vi "Write.vi"(8 "error in (no error)":errorcluster, 9 "Cell (Append to next row)":cluster{"Row":i32, "Col":i32}={"Row"=-1, "Col"=-1}, 10 "Data":variant, 11 "Excel in":refnum<class "Excel.lvclass">) -> (0 "error out":errorcluster, 3 "Excel out":refnum<class "Excel.lvclass">)   [LabVIEW 2016, in "Excel.lvclass"]
doc: "Writes Data to the active worksheet referenced in the Excel input object.\n\nIf a cell is specified and Data is a singleton the data will be written to that cell. \nIf a cell is specified and Data is 1D the data will be written beginning at that cell and continuing rightwards.\nIf a cell is specified and Data is 2D the data will be written as a matrix with it's first (top left) element beginning in that cell. The data will be formatted as it appears in LabVIEW (i.e. no transposition required).\n\nIf cell is not specified Data will be written starting from column A in the first available row following the rules outlined above.\n\nData cannot have dimension higher than 2."
uses:
  Excel.lvclass
  Excel.lvclass/Excel.ctl
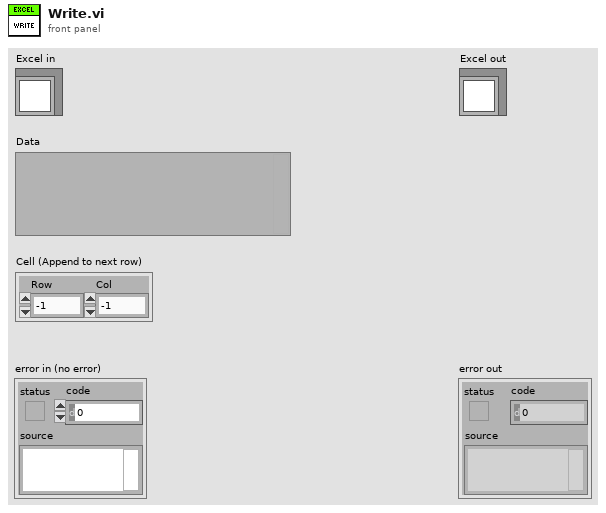
[diagram p1: front panel]
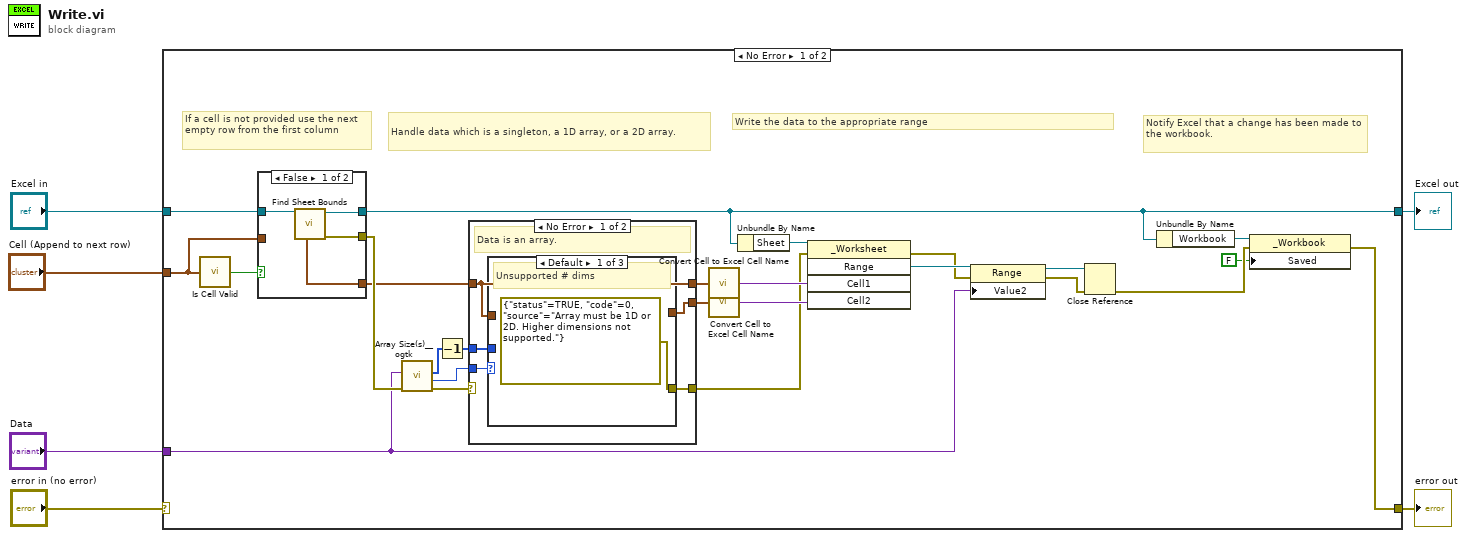
[diagram p0: block diagram]
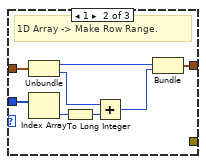
[diagram p2: hidden frame]
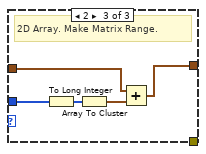
[diagram p3: hidden frame]
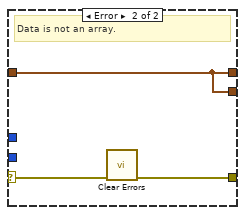
[diagram p4: hidden frame]
diagram:
  n1 = case shown="No Error" "error in (no error)" {
    selector: "error in (no error)" -> [_ w61]
    tunnel: [w7 w61] -> w5
    tunnel: [w10 w60] -> w3
    tunnel: "Excel in" -> [w24 w60]
    tunnel: "Data" -> [w19 _]
    tunnel: "Cell (Append to next row)" -> [w23 _]
    frame No Error {
      # "Notify Excel that a change has been made to the workbook."
      # "Write the data to the appropriate range"
      # "Handle data which is a singleton, a 1D array, or a 2D array."
      # "If a cell is not provided use the next empty row from the first column"
      n2 = call "Is Cell Valid.vi"("Cell"=w23) -> ("Valid?"=w25:bool)
      n3 = case shown="False" w25 {
        tunnel: w24 -> [w57 w59]
        tunnel: [w56 w59] -> w10
        tunnel: w23 -> [_ w58]
        tunnel: [w54 w58] -> w17
        tunnel: [w55 _] -> w20
        frame False {
          n4 = call "Find Sheet Bounds.vi"("Excel in"=w57) -> ("error out"=w55:errorcluster, "Excel out"=w56:refnum<class "Excel.lvclass">, "Bounding Row ++"=w54:cluster{"Row":i32, "Column":i32})  [unwired: 4 in, 4 out]
        }
        frame True {
        }
      }
      n5 = call <userlib>:"Array Size(s)__ogtk.vi"("error in (no error)"=w20, "Array"=w19) -> ("error out"=w21:errorcluster, "N dims"=w18:u32, "Size(s)"=w11:u32[])  [unwired: 7 in]
      n6 = Decrement(x=w11) -> (x-1=w12:u32[])
      n7 = case shown="No Error" w21 {
        selector: w21 -> [_ w53]
        tunnel: w12 -> [w34 _]
        tunnel: w18 -> [w36 _]
        tunnel: w17 -> [w33 w52]
        tunnel: [w33 w52] -> w16
        tunnel: [w32 w52] -> w15
        tunnel: [w35 w51] -> w13
        frame No Error {
          # "Data is an array."
          n8 = case shown="Default" w36 {
            tunnel: [errorcluster {"status"=TRUE, "code"=0, "source"="Array must be 1D or 2D. Higher dimensions not supported."} ("error constant") _ _] -> w35
            tunnel: w34 -> [_ w45 w50]
            tunnel: w33 -> [_ w44 w47]
            tunnel: [_ w40 w46] -> w32
            frame Default {
              # "Unsupported # dims"
            }
            frame 1 {
              # "1D Array -> Make Row Range."
              n9 = Unbundle(w44) -> ("Row"=w41:i32, "Col"=w43:i32)
              n10 = Index Array(array=w45) -> (element=w38:u32)  [unwired: 1 in]
              n11 = To Long Integer(number=w38) -> (32bit integer=w39:i32)
              n12 = Add(x=w43, y=w39) -> (x+y=w42:i32)
              n13 = Bundle("Row"=w41, w42) -> (w40:cluster{"Row":i32, i32})  [unwired: 1 in]
            }
            frame 2 {
              # "2D Array. Make Matrix Range."
              n14 = To Long Integer(number=w50) -> (32bit integer=w49:i32[])
              n15 = Array To Cluster(array=w49) -> (cluster=w48:cluster{"[0]":i32, "[1]":i32})
              n16 = Add(x=w47, y=w48) -> (x+y=w46:cluster{i32, i32})
            }
          }
        }
        frame Error {
          # "Data is not an array."
          n17 = call <vilib>:"Clear Errors.vi"("error in (no error)"=w53) -> ("error out"=w51:errorcluster)  [unwired: 5 in, 1 out]
        }
      }
      n18 = call "Convert Cell to Excel Cell Name.vi"("Cell"=w16) -> ("Cell Name"=w22:variant)
      n19 = call "Convert Cell to Excel Cell Name.vi"("Cell"=w15) -> ("Cell Name"=w14:variant)
      n20 = Unbundle By Name(w10) -> ("Sheet"=w30:refnum<k7>)
      n21 = invoke class="_Worksheet" method="Range"(reference=w30, error in=w13, "Cell1"=w22, "Cell2"=w14) -> (error out=w28:errorcluster, "Range"=w29:refnum<k7>)  [unwired: 1 in, 3 out]
      n22 = property class="Range"(reference=w29, error in=w28, "Value2"=w19) -> (reference out=w27:refnum<k7>, error out=w26:errorcluster)
      n23 = Close Reference(reference=w27, error in (no error)=w26) -> (error out=w31:errorcluster)
      n24 = Unbundle By Name(w10) -> ("Workbook"=w9:refnum<k7>)
      n25 = property class="_Workbook"(reference=w9, error in=w31, "Saved"=FALSE) -> (error out=w7:errorcluster)  [unwired: 1 out]
    }
    frame Error {
    }
  }
  "error out" <- w5
  "Excel out" <- w3
